vi "placeBoxNow.vi"() -> ()   [LabVIEW 2022 SP3]
panel:
  in  "String":string
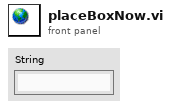
[diagram p1: front panel]
diagram:
